vi "Test Configuration Flatten.vi"() -> ()   [LabVIEW 2021]
uses:
  CIF_CIPC_Chan/Typedef/Buffer Configuration Data.ctl
  <vilib>/CIF Foundation/CIF Utilities/DataTypes/Flatten Unflatten/Flatten U32.vi
  <vilib>/CIF Foundation/CIF Utilities/DataTypes/Flatten Unflatten/Flatten I32.vi
  <vilib>/CIF Foundation/CIF Utilities/DataTypes/Flatten Unflatten/Unflatten U32.vi
  <vilib>/CIF Foundation/CIF Utilities/DataTypes/Flatten Unflatten/Unflatten I32.vi
  CIF_CIPC_Chan/CIF_CIPC_Chn.lvclass
panel:
  out "Pass":bool
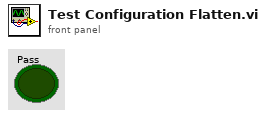
[diagram p1: front panel]
types:
  T1 = typedef "CIF_CIPC_Chn.lvclass/Buffer Configuration Data.ctl" = cluster{"Total Size":u32, "Read Size":u32, "Read Offset":u32, "Override CIPC Name":string, "Encoder Data":string}
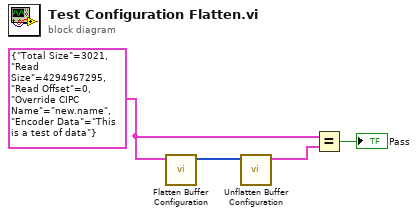
[diagram p0: block diagram]
diagram:
  w2 = T1 {"Total Size"=3021, "Read Size"=4294967295, "Read Offset"=0, "Override CIPC Name"="new.name", "Encoder Data"="This is a test of data"} ("Buffer Configuration")
  n1 = call "Flatten Buffer Configuration.vi"("Buffer Configuration"=w2) -> ("Flattened Configuration"=w4:u8[])  [unwired: 10 in]
  n2 = call "Unflatten Buffer Configuration.vi"("Flattened Configuration"=w4) -> ("Buffer Configuration"=w3:T1)  [unwired: 10 in]
  n3 = Equal?(x=w2, y=w3) -> (x = y?=→"Pass":bool)
